vi "APP_ByteToBit.vi"(0 "byte array":u8[](array[numeric])) -> (7 "bit array":i8[](array[numeric]))   [LabVIEW 2022 SP3]
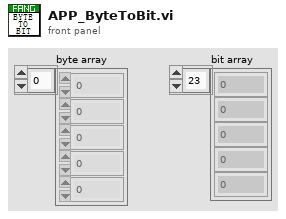
[diagram p1: front panel]
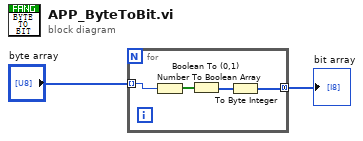
[diagram p0: block diagram]
diagram:
  n1 = for {
    tunnel: "byte array" -> [w6] mode=indexing
    tunnel: [w3] -> w2 mode=concatenating
    n2 = Number To Boolean Array(number=w6) -> (Boolean array=w5:bool[])
    n3 = Boolean To (0,1)(Boolean=w5) -> (0, 1=w4:i16[])
    n4 = To Byte Integer(number=w4) -> (8bit integer=w3:i8[])
  }
  "bit array" <- w2
